vi "0716206.vi"() -> ()   [LabVIEW 2021]
uses:
  <vilib>/Analysis/NI_AALBase.lvlib
panel:
  out "Clock":cluster{dbl[], dbl[]}[](graph)
  in  "stop":bool
  # "12"
  # "3"
  # "9"
  # "6"
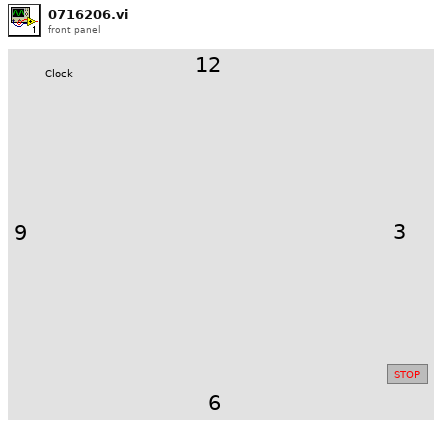
[diagram p1: front panel]
types:
  T1 = typedef "LVDateTimeRec.ctl" = cluster{"fractional second":dbl, "second":i32, "minute":i32, "hour":i32, "day of month":i32, "month":i32, "year":i32, "day of week":i32, "day of year":i32, "DST":i32}
  T2 = cluster{"Sinusoidal Pattern":dbl[], "Sinusoidal Pattern":dbl[]}
  T3 = cluster{"Sinusoidal Pattern":dbl[], "Sinusoidal Pattern":dbl[]}[]
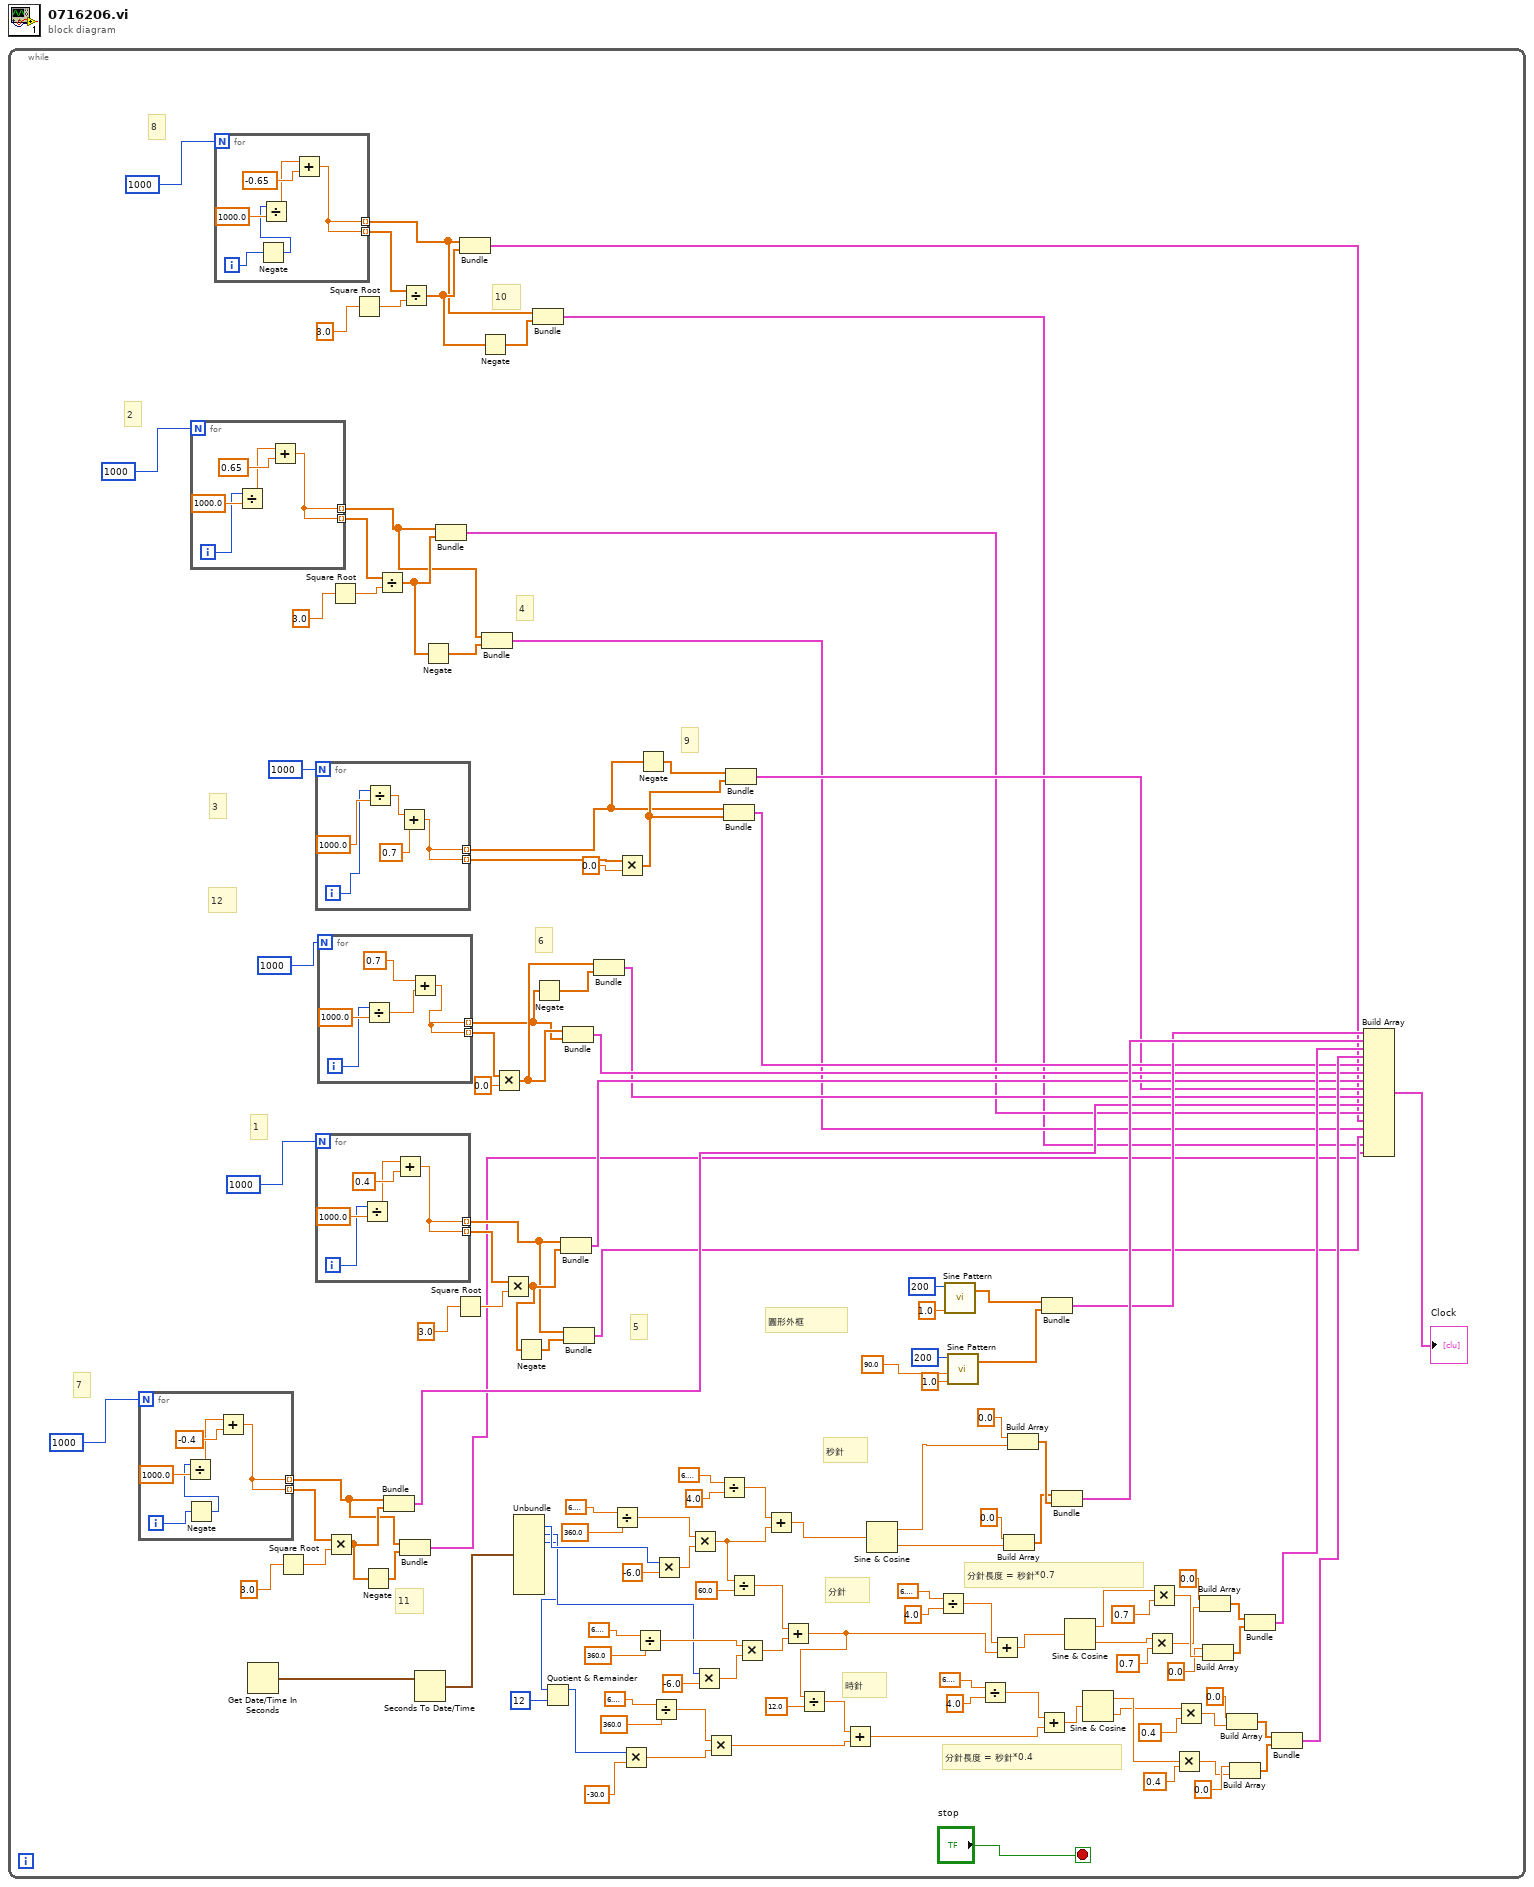
[diagram p0: block diagram]
diagram:
  n1 = while {
    stop <- "stop" stop-if-true
    # "11"
    # "10"
    # "9"
    # "6"
    # "5"
    # "4"
    # "8"
    # "2"
    # "7"
    # "1"
    # "3"
    # "12"
    # "圓形外框"
    # "分針長度 = 秒針*0.4"
    # "分針長度 = 秒針*0.7"
    # "時針"
    # "分針"
    # "秒針"
    n2 = for {
      N: 1000 -> [_]
      tunnel: [w148] -> w2 mode=indexing
      tunnel: [w148] -> w30 mode=indexing
      i -> [w147]
      n3 = Negate(x=w147) -> (-x=w146:i32)
      n4 = Divide(x=w146, y=1000.0) -> (x/y=w149:dbl)
      n5 = Add(x=w149, y=-0.4) -> (x+y=w148:dbl)
    }
    n6 = for {
      N: 1000 -> [_]
      tunnel: [w142] -> w14 mode=indexing
      tunnel: [w142] -> w24 mode=indexing
      i -> [w141]
      n7 = Divide(x=w141, y=1000.0) -> (x/y=w143:dbl)
      n8 = Add(x=w143, y=0.65) -> (x+y=w142:dbl)
    }
    n9 = for {
      N: 1000 -> [_]
      tunnel: [w137] -> w6 mode=indexing
      tunnel: [w137] -> w19 mode=indexing
      i -> [w136]
      n10 = Negate(x=w136) -> (-x=w135:i32)
      n11 = Divide(x=w135, y=1000.0) -> (x/y=w138:dbl)
      n12 = Add(x=w138, y=-0.65) -> (x+y=w137:dbl)
    }
    n13 = Get Date/Time In Seconds() -> (seconds since 1Jan1904=w134:timestamp)
    n14 = Square Root(x=3.0) -> (sqrt(x)=w28:dbl)
    n15 = for {
      N: 1000 -> [_]
      tunnel: [w162] -> w38 mode=indexing
      tunnel: [w162] -> w50 mode=indexing
      i -> [w165]
      n16 = Divide(x=w165, y=1000.0) -> (x/y=w163:dbl)
      n17 = Add(x=w163, y=0.7) -> (x+y=w162:dbl)
    }
    n18 = for {
      N: 1000 -> [_]
      tunnel: [w152] -> w10 mode=indexing
      tunnel: [w152] -> w45 mode=indexing
      i -> [w155]
      n19 = Divide(x=w155, y=1000.0) -> (x/y=w153:dbl)
      n20 = Add(x=w153, y=0.4) -> (x+y=w152:dbl)
    }
    n21 = for {
      N: 1000 -> [_]
      tunnel: [w157] -> w33 mode=indexing
      tunnel: [w157] -> w47 mode=indexing
      i -> [w160]
      n22 = Divide(x=w160, y=1000.0) -> (x/y=w158:dbl)
      n23 = Add(x=0.7, y=w158) -> (x+y=w157:dbl)
    }
    n24 = Multiply(x=w30, y=w28) -> (x*y=w4:dbl[])
    n25 = Square Root(x=3.0) -> (sqrt(x)=w23:dbl)
    n26 = Square Root(x=3.0) -> (sqrt(x)=w18:dbl)
    n27 = Negate(x=w4) -> (-x=w3:dbl[])
    n28 = Divide(x=w24, y=w23) -> (x/y=w16:dbl[])
    n29 = Bundle(w2, w4) -> (w27:cluster{dbl[], dbl[]})  [unwired: 1 in]
    n30 = Bundle(w2, w3) -> (w1:cluster{dbl[], dbl[]})  [unwired: 1 in]
    n31 = Divide(x=w19, y=w18) -> (x/y=w8:dbl[])
    n32 = Seconds To Date/Time(time stamp (now)=w134) -> (date time rec=w132:T1)  [unwired: 1 in]
    n33 = Negate(x=w16) -> (-x=w15:dbl[])
    n34 = Bundle(w14, w16) -> (w22:cluster{dbl[], dbl[]})  [unwired: 1 in]
    n35 = Square Root(x=3.0) -> (sqrt(x)=w43:dbl)
    n36 = Bundle(w6, w8) -> (w17:cluster{dbl[], dbl[]})  [unwired: 1 in]
    n37 = Negate(x=w8) -> (-x=w7:dbl[])
    n38 = Bundle(w14, w15) -> (w13:cluster{dbl[], dbl[]})  [unwired: 1 in]
    n39 = Multiply(x=w47, y=0.0) -> (x*y=w35:dbl[])
    n40 = Multiply(x=w45, y=w43) -> (x*y=w12:dbl[])
    n41 = Unbundle(w132) -> ("second"=w128:i32, "minute"=w108:i32, "hour"=w88:i32)  [unwired: 7 out]
    n42 = Negate(x=w12) -> (-x=w11:dbl[])
    n43 = Bundle(w6, w7) -> (w5:cluster{dbl[], dbl[]})  [unwired: 1 in]
    n44 = Negate(x=w33) -> (-x=w34:dbl[])
    n45 = Quotient & Remainder(x=w88, y=12) -> (x-y*floor(x/y)=w85:i32)  [unwired: 1 out]
    n46 = Bundle(w10, w12) -> (w40:cluster{dbl[], dbl[]})  [unwired: 1 in]
    n47 = Bundle(w35, w33) -> (w41:cluster{dbl[], dbl[]})  [unwired: 1 in]
    n48 = Bundle(w10, w11) -> (w9:cluster{dbl[], dbl[]})  [unwired: 1 in]
    n49 = Bundle(w35, w34) -> (w32:cluster{dbl[], dbl[]})  [unwired: 1 in]
    n50 = Divide(x=6.283185307179586, y=360.0) -> (x/y=w127:dbl)
    n51 = Multiply(x=w50, y=0.0) -> (x*y=w39:dbl[])
    n52 = Multiply(x=w85, y=-30.0) -> (x*y=w82:dbl)
    n53 = Divide(x=6.283185307179586, y=360.0) -> (x/y=w111:dbl)
    n54 = Negate(x=w38) -> (-x=w37:dbl[])
    n55 = Divide(x=6.283185307179586, y=360.0) -> (x/y=w81:dbl)
    n56 = Multiply(x=w128, y=-6.0) -> (x*y=w126:dbl)
    n57 = Multiply(x=w127, y=w126) -> (x*y=w116:dbl)
    n58 = Multiply(x=w108, y=-6.0) -> (x*y=w110:dbl)
    n59 = Multiply(x=w81, y=w82) -> (x*y=w77:dbl)
    n60 = Divide(x=6.283185307179586, y=4.0) -> (x/y=w123:dbl)
    n61 = Bundle(w38, w39) -> (w42:cluster{dbl[], dbl[]})  [unwired: 1 in]
    n62 = Bundle(w37, w39) -> (w36:cluster{dbl[], dbl[]})  [unwired: 1 in]
    n63 = Divide(x=w116, y=60.0) -> (x/y=w115:dbl)
    n64 = Multiply(x=w111, y=w110) -> (x*y=w114:dbl)
    n65 = Add(x=w123, y=w116) -> (x+y=w122:dbl)
    n66 = Add(x=w115, y=w114) -> (x+y=w79:dbl)
    n67 = Divide(x=w79, y=12.0) -> (x/y=w78:dbl)
    n68 = Add(x=w78, y=w77) -> (x+y=w73:dbl)
    n69 = Sine & Cosine(0:w122) -> (1:w120:dbl, 2:w121:dbl)
    n70 = Divide(x=6.283185307179586, y=4.0) -> (x/y=w105:dbl)
    n71 = call <vilib>:"Sine Pattern.vi"("cycles"=1.0, "samples"=200) -> ("Sinusoidal Pattern"=w56:dbl[])  [unwired: 2 in, 1 out]
    n72 = call <vilib>:"Sine Pattern.vi"("cycles"=1.0, "phase(degrees)"=90.0, "samples"=200) -> ("Sinusoidal Pattern"=w55:dbl[])  [unwired: 1 in, 1 out]
    n73 = Divide(x=6.283185307179586, y=4.0) -> (x/y=w74:dbl)
    n74 = Add(x=w105, y=w79) -> (x+y=w104:dbl)
    n75 = Build Array(0.0 ("element"), w121) -> (w91:dbl[])
    n76 = Build Array(0.0 ("element"), w120) -> (w92:dbl[])
    n77 = Add(x=w74, y=w73) -> (x+y=w72:dbl)
    n78 = Bundle("Sinusoidal Pattern"=w56, "Sinusoidal Pattern"=w55) -> (w53:T2)  [unwired: 1 in]
    n79 = Bundle(w91, w92) -> (w119:cluster{dbl[], dbl[]})  [unwired: 1 in]
    n80 = Sine & Cosine(0:w104) -> (1:w101:dbl, 2:w100:dbl)
    n81 = Sine & Cosine(0:w72) -> (1:w64:dbl, 2:w63:dbl)
    n82 = Multiply(x=w100, y=0.7) -> (x*y=w98:dbl)
    n83 = Multiply(x=w101, y=0.7) -> (x*y=w99:dbl)
    n84 = Multiply(x=w64, y=0.4) -> (x*y=w61:dbl)
    n85 = Multiply(x=w63, y=0.4) -> (x*y=w62:dbl)
    n86 = Build Array(0.0 ("element"), w98) -> (w94:dbl[])
    n87 = Build Array(0.0 ("element"), w99) -> (w95:dbl[])
    n88 = Build Array(0.0 ("element"), w62) -> (w66:dbl[])
    n89 = Build Array(0.0 ("element"), w61) -> (w67:dbl[])
    n90 = Bundle(w94, w95) -> (w93:cluster{dbl[], dbl[]})  [unwired: 1 in]
    n91 = Bundle(w66, w67) -> (w65:cluster{dbl[], dbl[]})  [unwired: 1 in]
    n92 = Build Array(w53, w119, w93, w65, w42, w41, w40, w36, w32, w27, w22, w17, w13, w9, w5, w1) -> (→"Clock":T3)
  }
